vi "UI_Config.vi"() -> ()   [LabVIEW 2016]
uses:
  <vilib>/Pansino Software/LabVIEW Architecture/Queue Management/PSARC_Queue Valid.vi
  <vilib>/Pansino Software/LabVIEW Architecture/Queue Management/PSARC_Queue Insert Element.vi
  <vilib>/Utility/error.llb/DialogType.ctl
  <vilib>/Pansino Software/LabVIEW Architecture/Queue Management/PSARC_Queue Destroy_Single.vi
  <vilib>/Pansino Software/LabVIEW Architecture/Queue Management/PSARC_Queue Remove Element.vi
  <vilib>/Pansino Software/ToolkitLib/Popup Toolkit/Private/Ctrls/PSPOP_Data Type.ctl
  <vilib>/Pansino Software/ToolkitLib/Popup Toolkit/Private/Ctrls/PSPOP_Grid.Cell Info.ctl
  <vilib>/Pansino Software/LabVIEW Architecture/Queue Management/PSARC_Queue Create_Single.vi
  <vilib>/Pansino Software/ToolkitLib/Popup Toolkit/Public/PSPOP_Popup Cluster.ctl
panel:
  out "Error Report":string
  in  "Popups":T1 {"Time" format="%<%Y/%m/%d %I:%M:%S>T"; "Boolean" items=["False", "True"]; "Ring" items=["100"=100, "200"=200, "500"=500, "1k"=1000, "2k"=2000, "5k"=5000, "10k"=10000, "20k"=20000, "40k"=40000]}
  in  "Tree":string(tree)
  in  "Caller":string
  # "Boolean Colors"
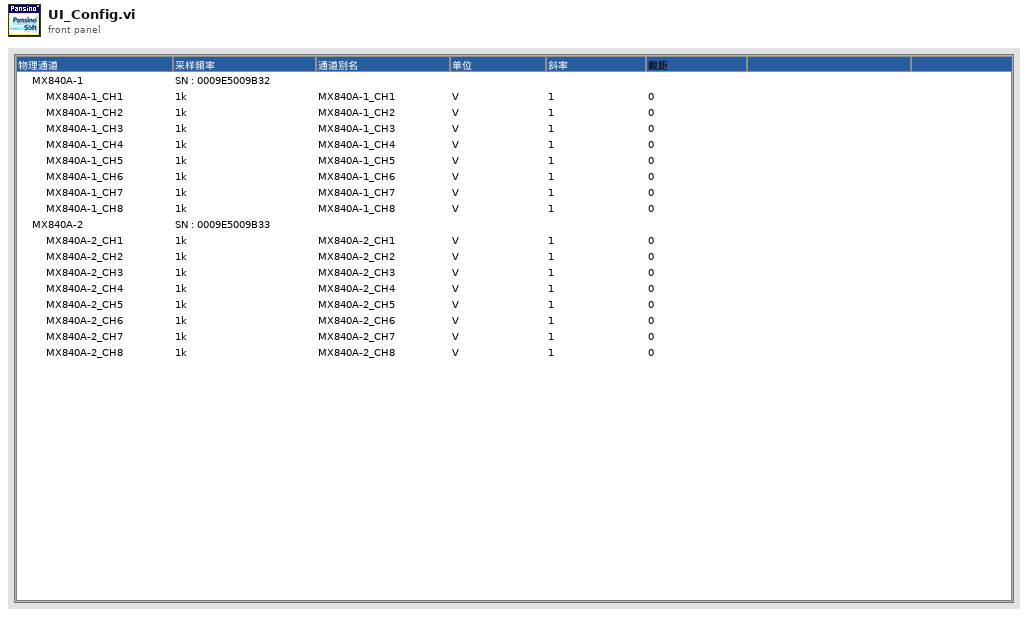
[diagram p1: front panel]
types:
  T1 = typedef "PSPOP_Popup Cluster.ctl" = cluster{"Unknown":bool, "Unknown 2":bool, "String":string, "Integer":i32, "Float":dbl, "Color":u32, "Boolean":u32, "Ring":u32, "Captioned String":cluster{"String":string, "OK":bool, "Cancel":bool}, "Captioned Integer":cluster{"First":i32, "OK":bool, "Cancel":bool}, "Boolean Colors":cluster{"False":cluster{"FG":u32, "BG":u32}, "True":cluster{"FG":u32, "BG":u32}, "T  to  F":cluster{"FG":u32, "BG":u32}, "F  to  T":cluster{"FG":u32, "BG":u32}, "OK":bool, "Cancel":bool}, "2-Int Cluster":cluster{"First":i32, "Second":i32, "OK":bool, "Cancel":bool}, "4-Int Cluster":cluster{"First":i32, "Second":i32, "Third":i32, "Fourth":i32, "OK":bool, "Cancel":bool}, "6-Dbl Cluster":cluster{"First":dbl, "Second":dbl, "Third":dbl, "Fourth":dbl, "Fourth 2":dbl, "Third 2":dbl, "OK":bool, "Cancel":bool}, "Path":path, "Combox":string, "Time":timestamp, "ShortCut":string}
  T2 = typedef "PSCHN_Card Para.ctl" = cluster{"Module Type":string, "Module Name":string, "ModuSN":string, "ModuIP":string, "Used?":bool, "Connected":bool, "Timing*":cluster{"Sample Rate":dbl}, "Channels":T3[]}
  T3 = typedef "PSCHN_Channel Para.ctl" = cluster{"CHTag*":string, "Used?*":bool, "CHName":string, "Unit":string, "斜率":dbl, "截距":dbl}
  T4 = cluster{"Error":errorcluster, "Exit":bool, "MainQ":cluster{"Main Queue":string, "Event":string, "Data":variant}, "PopUp Name":string, "All Ref":cluster{"Tree":refnum<vi>}, "PopUp Para":cluster{"ControlsRef":refnum<vi>, "Value":variant}, "Q-Caller":string, "Cards":T2[], "ConfigFilePath":path, "QXSystem reference":refnum<k24>, "QXDAQ reference":refnum<k24>}
  T5 = typedef "DialogType.ctl" = u16
  T6 = cluster{"TREE PNG":path, "User Guide":path, "DefaultSave":path, "BuildPath":path, "Image":path, "Modules":path, "Configuration":path, "License":path, "SplitFiles":path, "System.ini":path}
  T7 = cluster{"ControlsRef":refnum<vi>, "Value":variant}
  T8 = typedef "PSCFO_ParaDataType.ctl" = cluster{"ParaTag":string, "ParaName":string, "ParaType":string, "PicName":string, "ParaLevel":string, "DefaultValue":variant, "ParaVisable?":bool, "ParaOperation?":bool, "Operation":cluster{"ParaValue":string, "Operation":cluster{"ChangePara":cluster{"ParaName":string, "ParaData":string}[], "EnablePara":string[]}}[], "Ring Para":T9}
  T9 = typedef "PSLIST_Para Related.ctl" = cluster{"Strings":string[], "Values":ext[], "Use":bool, "Combox":string[], "Browse Options":T10, "Combo Box":cluster{"Allow Undefined Strings":bool}}
  T10 = typedef "LVBrowseOptionsTypeDef.ctl" = cluster{"Prompt":string, "Match Pattern":string, "Mode":enum32{"existing file", "new file", "new or existing file", "existing dir", "new dir", "new or existing dir", "existing file (use LLBs)", "new file (use LLBs)", "new or existing file (use LLBs)", "new or existing file or directory (use LLBs)", "existing dir (use LLBs)", "new dir (use LLBs)", "new or existing dir (use LLBs)", "existing file or dir", "new file or dir", "new or existing file or dir", "existing file or dir (use LLBs)", "new file or dir (use LLBs)"}, "Start Path":path, "Pattern Label":string, "Button Text":string}
  T11 = cluster{"Main Queue":string, "DAQ Queue":string, "ANA Queue":string, "CUI Queue":string, "Q-FocusList":string, "Q-Toolbar":string, "Q-Config":string}
  T12 = enum8{"Enabled", "Disabled", "Disabled and Grayed Out"}
  T13 = typedef "PSPOP_Grid.Cell Info.ctl" = cluster{"Tag":string, "Row":i32, "Column":i32, "In Symbol?":bool, "In Data?":bool, "Cell String":string, "Ctl Refnum":refnum<vi>, "Prop Type":T14, "Ring Strings":string[], "Ring Values":ext[], "New Cell String":string}
  T14 = typedef "PSPOP_Data Type.ctl" = enum16{"NO POPUP", "Unkown", "String", "Integer", "Float", "Color", "Boolean", "Ring", "Captioned String", "Captioned Integer", "Button Color", "2 Int Cluster", "4 Int Cluster", "6-Dbl Cluster", "Path", "Combox", "Time", "ShotCut String"}
  T15 = typedef "LVPoint32TypeDef.ctl" = cluster{"Horizontal":i32, "Vertical":i32}
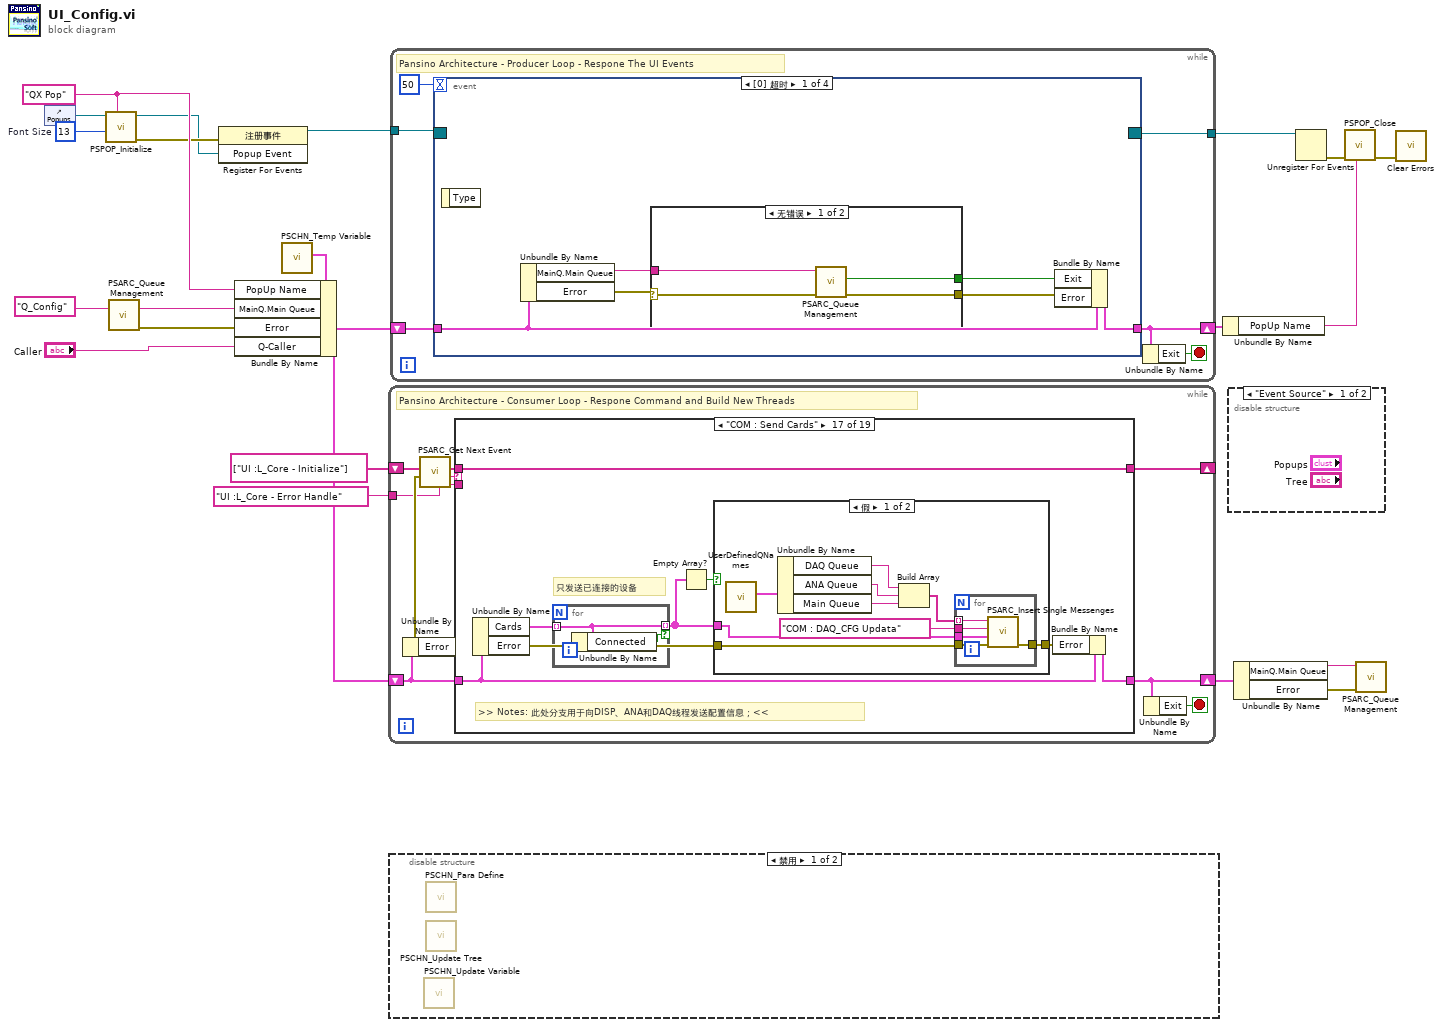
[diagram p0: block diagram]
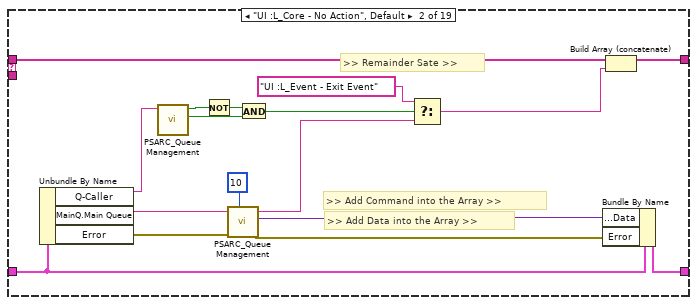
[diagram p5: hidden frame]
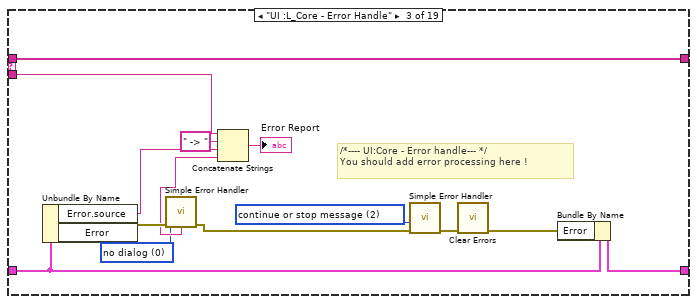
[diagram p6: hidden frame]
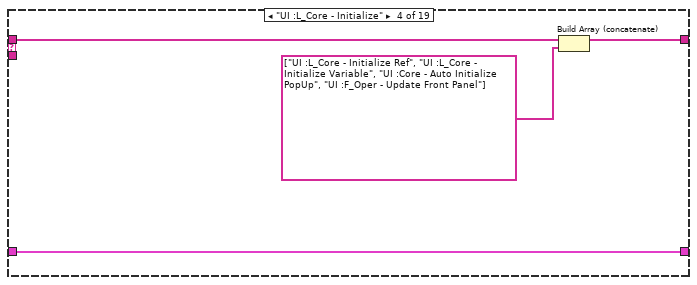
[diagram p7: hidden frame]
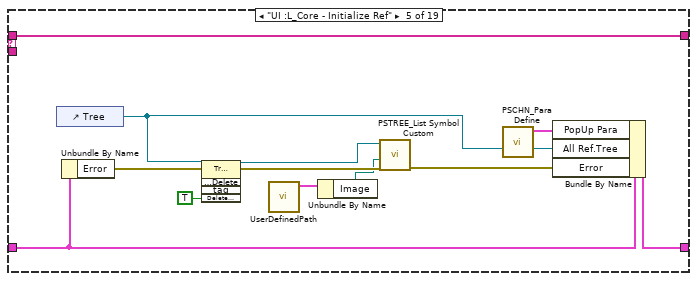
[diagram p8: hidden frame]
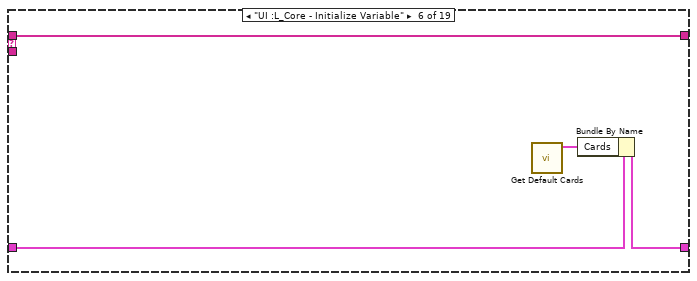
[diagram p9: hidden frame]
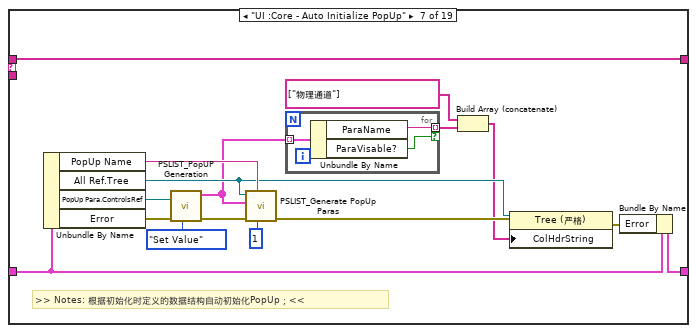
[diagram p10: hidden frame]
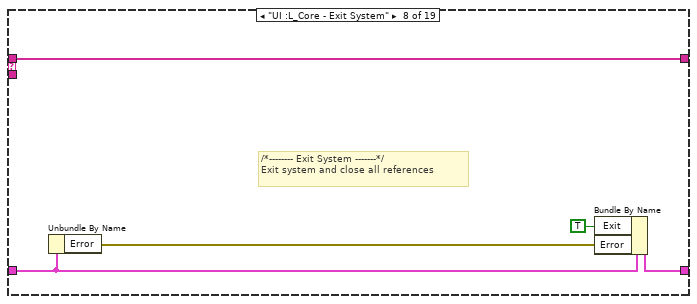
[diagram p11: hidden frame]
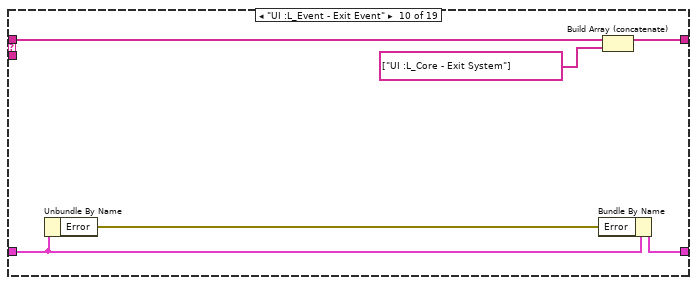
[diagram p13: hidden frame]
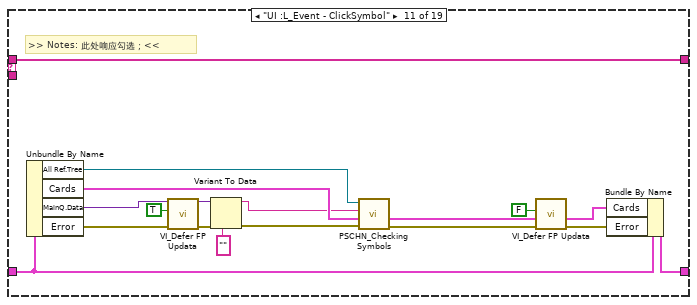
[diagram p14: hidden frame]
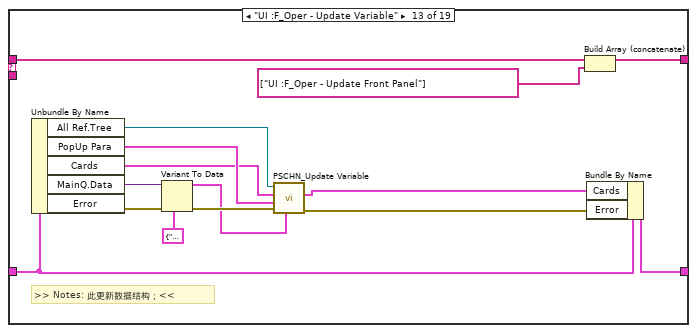
[diagram p16: hidden frame]
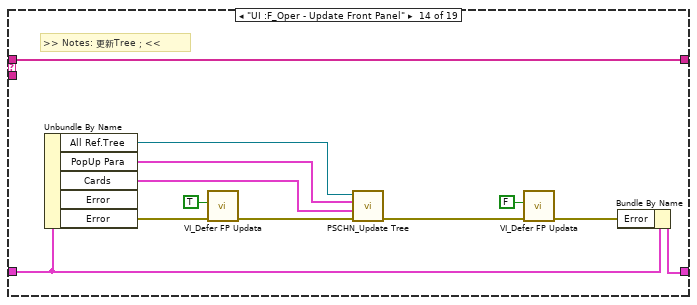
[diagram p17: hidden frame]
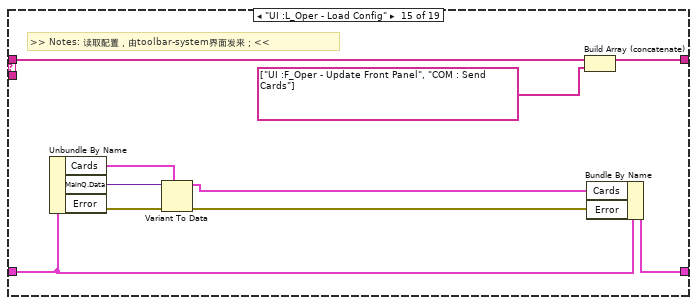
[diagram p18: hidden frame]
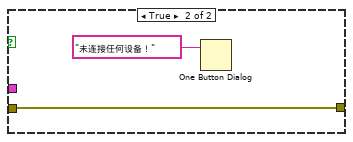
[diagram p20: hidden frame]
diagram:
  w2 = "Q_Config" ("MainQ.Main Queue")
  w17 = "QX Pop" ("Name")
  w12 = u32 13  # Font Size
  n1 = control-ref of="Popups"() -> (w14:refnum<vi>)
  n2 = call <vilib>:"PSPOP_Initialize.vi"("Name"=w17, "Font Size"=w12, "Popup Cluster Ref"=w14) -> ("error out"=w15:errorcluster, "Popup Event"=w13:refnum<user-event>)  [unwired: 7 in]
  n3 = call-poly <vilib>:"PSARC_Queue Management.vi"("Queue Name"=w2) -> ("error out"=w7:errorcluster)  [unwired: 9 in, 1 out]
  n4 = register-events(error in=w15, w13) -> (reference out=w16:refnum<event-registration>)  [unwired: 1 in, 1 out]
  n5 = call "PSCHN_Temp Variable.vi"() -> ("TempVariable"=w3:T4)  [unwired: 11 in]
  n6 = Bundle By Name(cluster=w3, "PopUp Name"=w17, "MainQ.Main Queue"=w2, "Error"=w7, "Q-Caller"="Caller") -> (w6:T4)
  n7 = while {
    shift-right: [w25] -> w11
    shift-left: w6 -> [w27]
    shift-right: [w28] -> _
    shift-left: string[] ["UI :L_Core - Initialize"] -> [w31]
    tunnel: "UI :L_Core - Error Handle" ("Error Handle") -> [w23]
    stop <- w24 stop-if-true
    # "Pansino Architecture - Consumer Loop - Respone Command and Build New Threads"
    n8 = Unbundle By Name(w27) -> ("Error"=w26:errorcluster)
    n9 = call <vilib>:"PSARC_Get Next Event.vi"("Error Handle"=w23, "error in (no error)"=w26, "event queue in"=w31) -> ("prev event"=w22:string, "next event"=w30:string, "event queue out"=w29:string[])  [unwired: 3 in]
    n10 = case shown="\"COM : Send Cards\"" w30 {
      tunnel: w27 -> [w33 w47 w62 w67 w78 w83 w99 w105 w109 w115 w131 w133 w148 w161 w170 w172 w180 w202 w219]
      tunnel: w29 -> [w32 w45 w64 w68 w80 w82 w100 w108 w110 w113 w117 w134 w149 w154 w171 w173 w181 w209 w212]
      tunnel: [w32 w44 w64 w66 w80 w82 w100 w108 w110 w112 w117 w134 w136 w154 w166 w173 w181 w209 w211] -> w28
      tunnel: [w33 w46 w63 w67 w79 w84 w98 w106 w109 w114 w130 w133 w147 w160 w169 w172 w179 w200 w218] -> w25
      tunnel: w22 -> [_ _ w52 _ _ _ _ _ _ _ _ _ _ _ _ _ _ _ _]
      frame "----------Core Status----------" {
      }
      frame "UI :L_Core - No Action", Default {
        # ">> Add Data into the Array >>"
        # ">> Add Command into the Array >>"
        # ">> Remainder Sate >>"
        n11 = Unbundle By Name(w47) -> ("Q-Caller"=w41:string, "MainQ.Main Queue"=w43:string, "Error"=w48:errorcluster)
        n12 = call-poly <vilib>:"PSARC_Queue Management.vi"("Queue Name(unamed)"=w41) -> ("Not Exist?"=w40:bool, "Empty Queue Name?"=w39:bool)  [unwired: 8 in, 1 out]
        n13 = Not(x=w39) -> (.not. x?=w38:bool)
        n14 = call-poly <vilib>:"PSARC_Queue Management.vi"("Time out(-1)_queue out"=10, "error in (no error)"=w48, "Queue Name(unamed)"=w43) -> ("error out"=w50:errorcluster, "Data"=w49:variant, "Event"=w36:string)  [unwired: 5 in, 1 out]
        n15 = And(x=w38, y=w40) -> (x .and. y?=w37:bool)
        n16 = Select(t="UI :L_Event - Exit Event" ("Event"), s=w37, f=w36) -> (s? t:f=w35:string)
        n17 = Bundle By Name(cluster=w47, "MainQ.Data"=w49, "Error"=w50) -> (w46:T4)
        n18 = Build Array (concatenate)(w45, w35) -> (w44:string[])
      }
      frame "UI :L_Core - Error Handle" {
        w51 = T5 0 items=["no dialog", "OK message", "continue or stop message", "OK message + warnings", "continue/stop + warnings"] ("type of dialog (OK msg:1)")
        w59 = T5 2 items=["no dialog", "OK message", "continue or stop message", "OK message + warnings", "continue/stop + warnings"] ("type of dialog (OK msg:1)")
        # "/*---- UI:Core - Error handle--- */\nYou should add error processing here !"
        n19 = Unbundle By Name(w62) -> ("Error.source"=w53:string, "Error"=w56:errorcluster)
        n20 = call <vilib>:"Simple Error Handler.vi"("type of dialog (OK msg:1)"=w51, "error in (no error)"=w56) -> ("error out"=w55:errorcluster, "message"=w54:string)  [unwired: 3 in, 3 out]
        n21 = Concatenate Strings(w52, " -> " ("字符串"), w53, w54) -> (→"Error Report":string)
        n22 = call <vilib>:"Simple Error Handler.vi"("type of dialog (OK msg:1)"=w59, "error in (no error)"=w55) -> ("error out"=w61:errorcluster)  [unwired: 3 in, 4 out]
        n23 = call <vilib>:"Clear Errors.vi"("error in (no error)"=w61) -> ("error out"=w60:errorcluster)  [unwired: 5 in, 1 out]
        n24 = Bundle By Name(cluster=w62, "Error"=w60) -> (w63:T4)
      }
      frame "UI :L_Core - Initialize" {
        n25 = Build Array (concatenate)(w68, string[] ["UI :L_Core - Initialize Ref", "UI :L_Core - Initialize Variable", "UI :Core - Auto Initialize PopUp", "UI :F_Oper - Update Front Panel"]) -> (w66:string[])
      }
      frame "UI :L_Core - Initialize Ref" {
        n26 = control-ref of="Tree"() -> (w73:refnum<vi>)
        n27 = Unbundle By Name(w78) -> ("Error"=w77:errorcluster)
        n28 = invoke class="Tree (严格)" method="Edit Tree Items.Delete"(reference=w73, error in=w77, "Delete Children"=TRUE ("删除子项？")) -> (reference out=w74:refnum<vi>, error out=w76:errorcluster)  [unwired: 2 in, 3 out]
        n29 = call "UserDefinedPath.vi"() -> ("UserDefinedPath"=w71:T6)  [unwired: 11 in]
        n30 = Unbundle By Name(w71) -> ("Image"=w70:path)
        n31 = call <vilib>:"PSTREE_List Symbol Custom.vi"("error in"=w76, "PicturePath"=w70, "ListRef"=w74) -> ("error out"=w75:errorcluster)  [unwired: 7 in, 1 out]
        n32 = call "PSCHN_Para Define.vi"() -> ("PopUp Para"=w72:T7)  [unwired: 11 in]
        n33 = Bundle By Name(cluster=w78, "PopUp Para"=w72, "All Ref.Tree"=w73, "Error"=w75) -> (w79:T4)
      }
      frame "UI :L_Core - Initialize Variable" {
        n34 = call "Get Default Cards.vi"() -> ("Cards"=w81:T2[])  [unwired: 11 in]
        n35 = Bundle By Name(cluster=w83, "Cards"=w81) -> (w84:T4)
      }
      frame "UI :Core - Auto Initialize PopUp" {
        # ">> Notes: 根据初始化时定义的数据结构自动初始化PopUp；<<"
        n36 = Unbundle By Name(w99) -> ("PopUp Name"=w94:string, "All Ref.Tree"=w92:refnum<vi>, "PopUp Para.ControlsRef"=w89:refnum<vi>, "Error"=w97:errorcluster)
        n37 = call <vilib>:"PSLIST_PopUP Generation.vi"("Commond"=enum16{"Set Value", "Get Value"}."Set Value", "错误输入（无错误）"=w97, "ControlsRef"=w89) -> ("error out"=w96:errorcluster, "PopUpPara"=w88:T8[])  [unwired: 7 in]
        n38 = call <vilib>:"PSLIST_Generate PopUp Paras.vi"("Begin Column"=1, "Name"=w94, "error in (no error)"=w96, "Parameter"=w88, "Ctl Refnum"=w92) -> ("error out"=w91:errorcluster)  [unwired: 6 in]
        n39 = for {
          tunnel: w88 -> [w103] mode=indexing
          tunnel: [w102] -> w87 mode=indexing if=w101
          n40 = Unbundle By Name(w103) -> ("ParaName"=w102:string, "ParaVisable?"=w101:bool)
        }
        n41 = Build Array (concatenate)(string[] ["物理通道"] ("array"), w87) -> (w86:string[])
        n42 = property class="Tree (严格)"(reference=w92, error in=w91, "ColHdrString"=w86) -> (error out=w90:errorcluster)  [unwired: 1 out]
        n43 = Bundle By Name(cluster=w99, "Error"=w90) -> (w98:T4)
      }
      frame "UI :L_Core - Exit System" {
        # "/*-------- Exit System -------*/\nExit system and close all references"
        n44 = Unbundle By Name(w105) -> ("Error"=w107:errorcluster)
        n45 = Bundle By Name(cluster=w105, "Exit"=TRUE, "Error"=w107) -> (w106:T4)
      }
      frame "----------Events----------" {
        # ">> Notes: 此处分支主要用于响应事件结构，考虑多个事件的合并，可在此处执行代码后进行界面刷新；<<"
      }
      frame "UI :L_Event - Exit Event" {
        n46 = Unbundle By Name(w115) -> ("Error"=w116:errorcluster)
        n47 = Bundle By Name(cluster=w115, "Error"=w116) -> (w114:T4)
        n48 = Build Array (concatenate)(w113, string[] ["UI :L_Core - Exit System"] ("数组")) -> (w112:string[])
      }
      frame "UI :L_Event - ClickSymbol" {
        # ">> Notes: 此处响应勾选；<<"
        n49 = Unbundle By Name(w131) -> ("All Ref.Tree"=w128:refnum<vi>, "Cards"=w127:T2[], "MainQ.Data"=w129:variant, "Error"=w124:errorcluster)
        n50 = call "VI_Defer FP Updata.vi"("error in"=w124, "Defer updata?"=TRUE) -> ("错误输出"=w123:errorcluster)  [unwired: 8 in, 1 out]
        n51 = Variant To Data(error in=w123, type="" ("Tag"), Variant=w129) -> (data=w125:string, error out=w132:errorcluster)
        n52 = call "PSCHN_Checking Symbols.vi"("error in (no error)"=w132, "Cards"=w127, "Tag"=w125, "CfgList Tree"=w128) -> ("error out"=w121:errorcluster, "Cards Out"=w118:T2[])  [unwired: 6 in]
        n53 = call "VI_Defer FP Updata.vi"("error in"=w121, "Defer updata?"=FALSE) -> ("错误输出"=w120:errorcluster)  [unwired: 8 in, 1 out]
        n54 = Bundle By Name(cluster=w131, "Cards"=w118, "Error"=w120) -> (w130:T4)
      }
      frame "----------Operations----------" {
        # ">> Notes: 此处分支主要用于数据结构相关操作，并考虑复用；<<"
      }
      frame "UI :F_Oper - Update Variable" {
        # ">> Notes: 此更新数据结构；<<"
        n55 = Unbundle By Name(w148) -> ("All Ref.Tree"=w140:refnum<vi>, "PopUp Para"=w139:T7, "Cards"=w137:T2[], "MainQ.Data"=w145:variant, "Error"=w146:errorcluster)
        n56 = Variant To Data(error in=w146, type=cluster{"Tag":string, "Popup Value":variant} {"Tag"="", "Popup Value"=variant} ("output cluster"), Variant=w145) -> (data=w138:cluster{"Tag":string, "Popup Value":variant}, error out=w143:errorcluster)
        n57 = call "PSCHN_Update Variable.vi"("data"=w138, "error in (no error)"=w143, "PopUp Para"=w139, "Cards"=w137, "Tree"=w140) -> ("error out"=w142:errorcluster, "Cards Out"=w141:T2[])  [unwired: 5 in]
        n58 = Build Array (concatenate)(w149, string[] ["UI :F_Oper - Update Front Panel"]) -> (w136:string[])
        n59 = Bundle By Name(cluster=w148, "Cards"=w141, "Error"=w142) -> (w147:T4)
      }
      frame "UI :F_Oper - Update Front Panel" {
        # ">> Notes: 更新Tree；<<"
        n60 = Unbundle By Name(w161) -> ("All Ref.Tree"=w159:refnum<vi>, "PopUp Para"=w158:T7, "Cards"=w157:T2[], "Error"=w151:errorcluster)  [unwired: 1 out]
        n61 = call "VI_Defer FP Updata.vi"("error in"=w151, "Defer updata?"=TRUE) -> ("错误输出"=w150:errorcluster)  [unwired: 8 in, 1 out]
        n62 = call "PSCHN_Update Tree.vi"("error in (no error)"=w150, "Cards"=w157, "PopUp Para"=w158, "Tree"=w159) -> ("error out"=w153:errorcluster)  [unwired: 7 in]
        n63 = call "VI_Defer FP Updata.vi"("error in"=w153, "Defer updata?"=FALSE) -> ("错误输出"=w152:errorcluster)  [unwired: 8 in, 1 out]
        n64 = Bundle By Name(cluster=w161, "Error"=w152) -> (w160:T4)
      }
      frame "UI :L_Oper - Load Config" {
        # ">> Notes: 读取配置，由toolbar-system界面发来；<<"
        n65 = Unbundle By Name(w170) -> ("Cards"=w163:T2[], "MainQ.Data"=w167:variant, "Error"=w168:errorcluster)
        n66 = Variant To Data(error in=w168, type=w163, Variant=w167) -> (data=w162:T2[], error out=w164:errorcluster)
        n67 = Build Array (concatenate)(w171, string[] ["UI :F_Oper - Update Front Panel", "COM : Send Cards"]) -> (w166:string[])
        n68 = Bundle By Name(cluster=w170, "Cards"=w162, "Error"=w164) -> (w169:T4)
      }
      frame "----------Communication----------" {
        # ">> Notes: 此处分支主要用于与其他线程通信，如无，可以删除；<<"
      }
      frame "COM : Send Cards" {
        # "只发送已连接的设备"
        # ">> Notes: 此处分支用于向DISP、ANA和DAQ线程发送配置信息；<<"
        n69 = Unbundle By Name(w180) -> ("Cards"=w176:T2[], "Error"=w177:errorcluster)
        n70 = for {
          tunnel: w176 -> [w199] mode=indexing
          tunnel: [w199] -> w174 mode=indexing if=w198
          n71 = Unbundle By Name(w199) -> ("Connected"=w198:bool)
        }
        n72 = Empty Array?(array=w174) -> (empty?=w175:bool)
        n73 = case shown="假" w175 {
          tunnel: [w190 w196] -> w178
          tunnel: w177 -> [w189 w196]
          tunnel: w174 -> [w182 _]
          frame False {
            n74 = call "UserDefinedQNames.vi"() -> ("All Queues"=w186:T11)  [unwired: 11 in]
            n75 = Unbundle By Name(w186) -> ("DAQ Queue"=w183:string, "ANA Queue"=w184:string, "Main Queue"=w187:string)
            n76 = Build Array(w183, w184, w187) -> (w188:string[])
            n77 = for {
              tunnel: [w194] -> w190
              tunnel: w188 -> [w192] mode=indexing
              tunnel: w182 -> [w191]
              tunnel: "COM : DAQ_CFG Updata" ("Event") -> [w193]
              tunnel: w189 -> [w195]
              n78 = call <vilib>:"PSARC_Insert Single Messenges.vi"("error in (no error)"=w195, "Data"=w191, "Order"=w193, "Queue Name"=w192) -> ("error out"=w194:errorcluster)  [unwired: 7 in]
            }
          }
          frame True {
            n79 = One Button Dialog(message="未连接任何设备！") -> ()  [unwired: 1 in, 1 out]
          }
        }
        n80 = Bundle By Name(cluster=w180, "Error"=w178) -> (w179:T4)
      }
      frame "COM : Request Cards" {
        # "将Cards信息发送给请求的线程"
        n81 = Unbundle By Name(w202) -> ("Cards"=w203:T2[], "MainQ.Main Queue"=w206:string, "MainQ.Data"=w208:variant, "Error"=w207:errorcluster)
        n82 = Variant To Data(error in=w207, type=w206, Variant=w208) -> (data=w204:string, error out=w205:errorcluster)
        n83 = call <vilib>:"PSARC_Insert Single Messenges.vi"("error in (no error)"=w205, "Data"=w203, "Queue Name"=w204) -> ("error out"=w201:errorcluster)  [unwired: 8 in]
        n84 = Bundle By Name(cluster=w202, "Error"=w201) -> (w200:T4)
      }
      frame "COM : Receive DevsInfo" {
        # "COM : Send Cards"
        # "DAQ线程发来设备信息"
        n85 = Unbundle By Name(w219) -> ("Cards"=w214:T2[], "MainQ.Data"=w221:variant, "Error"=w220:errorcluster)
        n86 = Variant To Data(error in=w220, type=w214, Variant=w221) -> (data=w217:T2[], error out=w216:errorcluster)
        n87 = call "Updata Cards by DevsInfo.vi"("error in (no error)"=w216, "DevsInfo"=w217, "Cards in"=w214) -> ("error out"=w215:errorcluster, "Cards out"=w213:T2[])  [unwired: 7 in]
        n88 = Bundle By Name(cluster=w219, "Cards"=w213, "Error"=w215) -> (w218:T4)
        n89 = Build Array (concatenate)(w212, string[] ["UI :F_Oper - Update Front Panel"] ("数组")) -> (w211:string[])
      }
    }
    n90 = Unbundle By Name(w25) -> ("Exit"=w24:bool)
  }
  n91 = disable-structure shown="禁用" {
    frame Disabled {
      n92 = call "PSCHN_Update Variable.vi"() -> ()  [unwired: 10 in, 2 out]
      n93 = call "PSCHN_Para Define.vi"() -> ()  [unwired: 11 in, 1 out]
      n94 = call "PSCHN_Update Tree.vi"() -> ()  [unwired: 11 in, 1 out]
    }
    frame Enabled {
    }
  }
  n95 = while {
    shift-right: [w225] -> w20
    shift-left: w6 -> [w226]
    tunnel: w16 -> [w223]
    tunnel: [w222] -> w19
    stop <- w224 stop-if-true
    # "Pansino Architecture - Producer Loop - Respone The UI Events"
    n96 = event shown="[0] 超时" {
      selector: w223 -> [_ _ _ _]
      dyn-events: [_ _ _ _] -> w222
      timeout: 50 -> [_ _ _ _]
      tunnel: w226 -> [w231 w242 w250 w283]
      tunnel: [w233 w241 w249 w281] -> w225
      event Timeout {
        n97 = event-data() -> ()  [unwired: 1 in, 1 out]
        n98 = Unbundle By Name(w231) -> ("MainQ.Main Queue"=w230:string, "Error"=w229:errorcluster)
        n99 = case shown="无错误" w229 {
          selector: w229 -> [w235 _]
          tunnel: [w237 _] -> w232
          tunnel: w230 -> [w236 _]
          tunnel: [w234 _] -> w228
          frame No Error {
            n100 = call-poly <vilib>:"PSARC_Queue Management.vi"("error in (no error)"=w235, "Queue Name(unamed)"=w236) -> ("error out"=w234:errorcluster, "Not Exist?"=w237:bool)  [unwired: 7 in, 1 out]
          }
          frame Error {
          }
        }
        n101 = Bundle By Name(cluster=w231, "Exit"=w232, "Error"=w228) -> (w233:T4)
      }
      event Panel Close? {
        n102 = event-data() -> ()  [unwired: 1 in, 1 out]
        n103 = Unbundle By Name(w242) -> ("MainQ.Main Queue"=w239:string, "Error"=w243:errorcluster)
        n104 = call-poly <vilib>:"PSARC_Queue Management.vi"("error in (no error)"=w243, "Event"="UI :L_Event - Exit Event", "Queue Name(unamed)"=w239) -> ("error out"=w240:errorcluster)  [unwired: 7 in, 1 out]
        n105 = Bundle By Name(cluster=w242, "Error"=w240) -> (w241:T4)
        n106 = event-data("Discard?"=TRUE ("放弃？")) -> ()  [unwired: 1 in, 1 out]
      }
      event "Tree": Mouse Down? {
        n107 = event-data() -> ("Button"=w246:u16, "CtlRef"=w248:refnum<vi>, "Coords"=w247:T15)  [unwired: 1 in]
        n108 = Unbundle By Name(w250) -> ("PopUp Name"=w245:string, "MainQ.Main Queue"=w255:string, "Error"=w253:errorcluster)
        n109 = Equal?(x=u16 1, y=w246) -> (x = y?=w251:bool)
        n110 = case shown="真" w251 {
          tunnel: w248 -> [_ w263]
          tunnel: w247 -> [_ w265]
          tunnel: [w258 w268] -> w256
          tunnel: w255 -> [_ w267]
          tunnel: [variant ("Variant") w266] -> w254
          tunnel: w253 -> [w258 w264]
          tunnel: w245 -> [_ w259]
          frame False {
          }
          frame True {
            n111 = property class="Tree (严格)"(reference=w263) -> ("DisabledEnum"=w262:T12)  [unwired: 1 in, 2 out]
            n112 = Equal?(x=T12."Enabled", y=w262) -> (x = y?=w260:bool)
            n113 = case shown="真" w260 {
              tunnel: [w269 w274] -> w268
              tunnel: w267 -> [_ w270]
              tunnel: [_ variant ("Variant")] -> w266
              tunnel: w265 -> [_ w273]
              tunnel: w264 -> [w269 w275]
              tunnel: w263 -> [_ w272]
              tunnel: w259 -> [_ w271]
              frame False {
              }
              frame True {
                n114 = call "PSCHN_JudgeClick.vi"("Coords"=w273, "Error In (no error)"=w275, "Q_Name"=w270, "PopUp Name"=w271, "TreeRef"=w272) -> ("Error Out"=w274:errorcluster)  [unwired: 6 in]
              }
            }
          }
        }
        n115 = Bundle By Name(cluster=w250, "MainQ.Data"=w254, "Error"=w256) -> (w249:T4)
        n116 = event-data() -> ()  [unwired: 2 in, 1 out]
      }
      event User Event {
        # ">> Notes: 此处发送数据结构更新指令，如有必要，随后更新前面板；<<"
        n117 = event-data() -> ("Valid?"=w288:bool, "Popup Value"=w286:variant, "Call Data"=w287:variant)  [unwired: 1 in, 1 out]
        n118 = Unbundle By Name(w283) -> ("MainQ.Main Queue"=w280:string, "Error"=w285:errorcluster)
        n119 = Variant To Data(error in=w285, type=T13 {"Tag"="", "Row"=0, "Column"=0, "In Symbol?"=FALSE, "In Data?"=FALSE, "Cell String"="", "Ctl Refnum"=refnum, "Prop Type"=enum."Unkown", "Ring Strings"=[], "Ring Values"=[], "New Cell String"=""} ("Cell Info (type only)"), Variant=w287) -> (data=w292:T13, error out=w284:errorcluster)
        n120 = Unbundle By Name(w292) -> ("Tag"=w278:string, "Row"=w291:i32)
        n121 = Equal?(x=w291, y=-1) -> (x = y?=w289:bool)
        n122 = case shown="假" w289 {
          tunnel: w288 -> [w300 _]
          tunnel: w286 -> [w299 _]
          tunnel: w287 -> [w298 _]
          tunnel: w284 -> [w297 w313]
          tunnel: [w296 w313] -> w282
          tunnel: w280 -> [w295 _]
          tunnel: "UI :F_Oper - Update Variable" -> [w294 _]
          tunnel: w278 -> [w293 _]
          frame False {
            n123 = case shown="真" w300 {
              tunnel: w299 -> [_ w303]
              tunnel: w298 -> [_ w307]
              tunnel: w297 -> [w301 w312]
              tunnel: [w301 w310] -> w296
              tunnel: w295 -> [_ w309]
              tunnel: w294 -> [_ w308]
              tunnel: w293 -> [_ w304]
              frame False {
              }
              frame True {
                n124 = call <vilib>:"PSPOP_Update Cell String.vi"("error in (no error)"=w312, "Call Data (must be Cell Info cluster)"=w307, "Popup Value"=w303) -> ("error out"=w311:errorcluster, "Cell Data"=w302:variant)  [unwired: 7 in]
                n125 = Bundle("Tag"=w304, "Cell Data"=w302) -> (w305:cluster{"Tag":string, "Cell Data":variant})  [unwired: 1 in]
                n126 = To Variant(anything=w305) -> (Variant=w306:variant)
                n127 = call-poly <vilib>:"PSARC_Queue Management.vi"("error in (no error)"=w311, "Data"=w306, "Event"=w308, "Queue Name(unamed)"=w309) -> ("error out"=w310:errorcluster)  [unwired: 6 in, 1 out]
              }
            }
          }
          frame True {
          }
        }
        n128 = Bundle By Name(cluster=w283, "Error"=w282) -> (w281:T4)
      }
    }
    n129 = Unbundle By Name(w225) -> ("Exit"=w224:bool)
  }
  n130 = Unbundle By Name(w20) -> ("PopUp Name"=w21:string)
  n131 = disable-structure shown="\"Event Source\"" {
    frame condition #0 (active) {
    }
    frame condition #1 {
    }
  }
  n132 = Unbundle By Name(w11) -> ("MainQ.Main Queue"=w8:string, "Error"=w10:errorcluster)
  n133 = Unregister For Events(event registration refnum=w19) -> (error out=w18:errorcluster)  [unwired: 1 in]
  n134 = call <vilib>:"PSPOP_Close.vi"("Name"=w21, "error in (no error)"=w18) -> ("error out"=w1:errorcluster)  [unwired: 9 in]
  n135 = call-poly <vilib>:"PSARC_Queue Management.vi"("error in (no error)"=w10, "Queue Name(unamed)"=w8) -> ()  [unwired: 7 in, 3 out]
  n136 = call <vilib>:"Clear Errors.vi"("error in (no error)"=w1) -> ()  [unwired: 5 in, 2 out]
